vi "SupportedMeasurementType.vi"(8 "error in (no error)":errorcluster, 11 "ChromaAcLoad in":refnum<class "ChromaAcLoad.lvclass">) -> (0 "error out":errorcluster, 3 "ChromaAcLoad out":refnum<class "ChromaAcLoad.lvclass">)   [LabVIEW 2018, in "AcPwrPlugins.lvlib" / "ChromaAcLoad.lvclass"]
doc: "This VI checks if Measurment Types selected are capable by the instrument based on the instruments configuration."
uses:
  ChromaAcLoad.lvclass
  TypeDefs/MeasurementType.ctl
  <vilib>/Utility/error.llb/Error Cluster From Error Code.vi
  <vilib>/ErrorRing/Error Ring.xnode
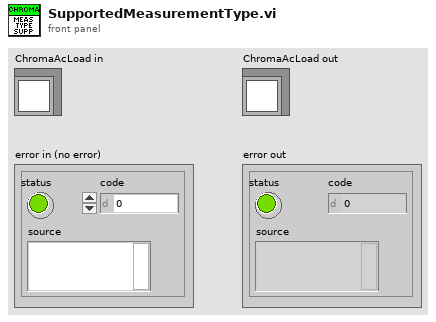
[diagram p1: front panel]
types:
  T1 = typedef "AcPwrPlugins.lvlib/ChromaAcLoad.lvclass/Device(s)Settings.ctl" = cluster{"Configuration Mode":enum16{"Constant Voltage (DC)", "Constant Power (DC)", "Constant Power (AC)", "Constant Current (DC)", "Constant Current (AC)", "Constant Resistance (DC)", "Constant Resistance (AC)", "Rectified Mode (DC)", "Inrush (AC)", "RLC CP (AC)", "RLC (AC)"}, "Phases":cluster{"Handle":string, "Name":string, "Phase Select":i32, "Instrument Options":string, "id query (T)":bool, "reset device (T)":bool, "Load Short Circuited":bool, "Line Synchronization":bool, "Load Current (A/Arms)":dbl, "Load Voltage (V/Vrms)":dbl, "Load Power (W)":dbl, "Load Resistance (Ohms)":dbl, "Load Current Peak Limit (A)":dbl, "Load Current Limit (A/Arms)":dbl, "Load Power Limit (W)":dbl, "Synch Frequency (Hz)":dbl, "Priority":enum16{"CF Only", "PF Only", "Both (CF)", "Both (PF)"}, "Crest Factor":dbl, "Power Factor":dbl, "Slew Rate":cluster{"Rise Slew Rate (A/ms)":i32, "Fall Slew Rate (A/ms)":i32}, "LC/RLC Mode":cluster{"Capacitance (uF)":i32, "Inductance (uH)":i32, "Series Resistance (Ohm)":dbl, "Parallel Resistance (Ohm)":dbl}, "Timing":cluster{"TimingOn":enum16{""}, "Hours":u32, "Minutes":u32, "Seconds":dbl, "CutoffVoltage":dbl}, "Connected":bool}[], "MeasName":string}
  T2 = typedef "AcPwrPlugins.lvlib/ChromaAcLoad.lvclass/Measurements.ctl" = cluster{"Handle":string, "Name":string, "Enabled":bool, "Measurement Value":dbl, "Hold Peak Current Measurement":bool, "btnMeasFetch":bool, "ProtectionStatusString":string, "Measurement Type":T3}[]
  T3 = typedef "AcPwrPlugins.lvlib/ChromaAcLoad.lvclass/MeasurementType.ctl" = enum16{"Voltage (Vrms or V)", "Current (Arms or A)", "Power (W)", "Peak Voltage (V)", "Peak Current (A)", "Peak Power (W)", "Frequency (Hz)", "Resistance (Ohms)", "Voltage Overshoot (V)", "Positive Peak Current (A)", "Voltage Undershoot (V)", "Negative Peak Current (A)", "Apparent Power (VA)", "Reacitive Power (VAR)", "Voltage THD", "Power Factor", "Current's Crest Factor"}
  T4 = cluster{"Handle":string, "Name":string, "Phase Select":i32, "Instrument Options":string, "id query (T)":bool, "reset device (T)":bool, "Load Short Circuited":bool, "Line Synchronization":bool, "Load Current (A/Arms)":dbl, "Load Voltage (V/Vrms)":dbl, "Load Power (W)":dbl, "Load Resistance (Ohms)":dbl, "Load Current Peak Limit (A)":dbl, "Load Current Limit (A/Arms)":dbl, "Load Power Limit (W)":dbl, "Synch Frequency (Hz)":dbl, "Priority":enum16{"CF Only", "PF Only", "Both (CF)", "Both (PF)"}, "Crest Factor":dbl, "Power Factor":dbl, "Slew Rate":cluster{"Rise Slew Rate (A/ms)":i32, "Fall Slew Rate (A/ms)":i32}, "LC/RLC Mode":cluster{"Capacitance (uF)":i32, "Inductance (uH)":i32, "Series Resistance (Ohm)":dbl, "Parallel Resistance (Ohm)":dbl}, "Timing":cluster{"TimingOn":enum16{""}, "Hours":u32, "Minutes":u32, "Seconds":dbl, "CutoffVoltage":dbl}, "Connected":bool}[]
  T5 = enum16{"Constant Voltage (DC)", "Constant Power (DC)", "Constant Power (AC)", "Constant Current (DC)", "Constant Current (AC)", "Constant Resistance (DC)", "Constant Resistance (AC)", "Rectified Mode (DC)", "Inrush (AC)", "RLC CP (AC)", "RLC (AC)"}
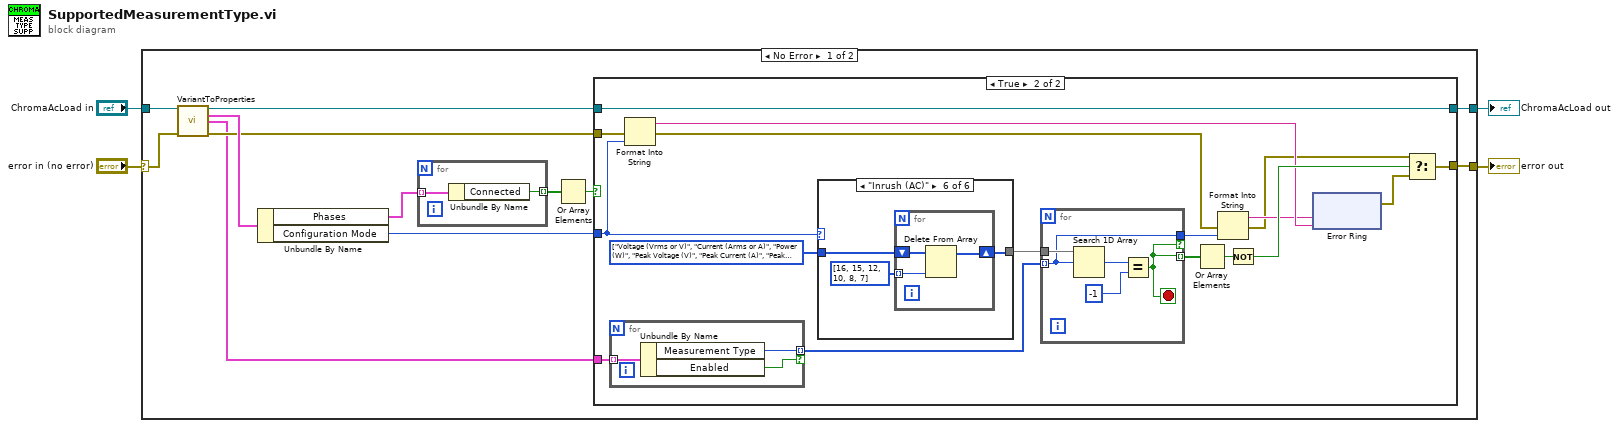
[diagram p0: block diagram]
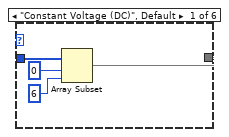
[diagram p3: hidden frame]
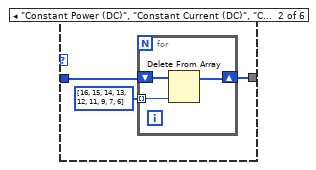
[diagram p4: hidden frame]
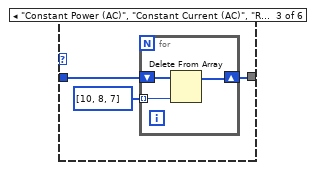
[diagram p5: hidden frame]
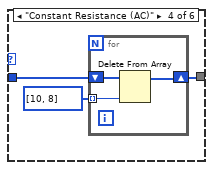
[diagram p6: hidden frame]
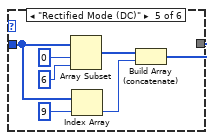
[diagram p7: hidden frame]
diagram:
  n1 = case shown="No Error" "error in (no error)" {
    selector: "error in (no error)" -> [w15 w90]
    tunnel: [w14 w90] -> w3
    tunnel: [w6 w89] -> w1
    tunnel: "ChromaAcLoad in" -> [w16 w89]
    frame No Error {
      n2 = call "VariantToProperties.vi"("ChromaAcLoad"=w16, "error in (no error)"=w15) -> ("ChromaAcLoad"=w7:refnum<class "ChromaAcLoad.lvclass">, "Device Properties"=w9:T1, "Meas"=w5:T2, "error out"=w8:errorcluster)  [unwired: 7 in, 3 out]
      n3 = Unbundle By Name(w9) -> ("Phases"=w12:T4, "Configuration Mode"=w13:T5)
      n4 = for {
        tunnel: w12 -> [w18] mode=indexing
        tunnel: [w17] -> w11 mode=indexing
        n5 = Unbundle By Name(w18) -> ("Connected"=w17:bool)
      }
      n6 = Or Array Elements(Boolean array=w11) -> (logical OR=w10:bool)
      n7 = case shown="True" w10 {
        tunnel: w5 -> [_ w36]
        tunnel: [w20 w29] -> w14
        tunnel: w13 -> [_ w28]
        tunnel: w8 -> [w20 w22]
        tunnel: w7 -> [w19 w21]
        tunnel: [w19 w21] -> w6
        frame False {
        }
        frame True {
          w37 = T3[] [enum."Voltage (Vrms or V)", enum."Current (Arms or A)", enum."Power (W)", enum."Peak Voltage (V)", enum."Peak Current (A)", enum."Peak Power (W)", enum."Frequency (Hz)", enum."Resistance (Ohms)", enum."Voltage Overshoot (V)", enum."Positive Peak Current (A)", enum."Voltage Undershoot (V)", enum."Negative Peak Current (A)", enum."Apparent Power (VA)", enum."Reacitive Power (VAR)", enum."Voltage THD", enum."Power Factor", enum."Current's Crest Factor"] items=["Voltage (Vrms or V)", "Current (Arms or A)", "Power (W)", "Peak Voltage (V)", "Peak Current (A)", "Peak Power (W)", "Frequency (Hz)", "Resistance (Ohms)", "Voltage Overshoot (V)", "Positive Peak Current (A)", "Voltage Undershoot (V)", "Negative Peak Current (A)", "Apparent Power (VA)", "Reacitive Power (VAR)", "Voltage THD", "Power Factor", "Current's Crest Factor"] ("MeasurementTypeArray")
          n8 = for {
            tunnel: w36 -> [w88] mode=indexing
            tunnel: [w87] -> w35 mode=indexing if=w86
            n9 = Unbundle By Name(w88) -> ("Measurement Type"=w87:T3, "Enabled"=w86:bool)
          }
          n10 = Format Into String(error in=w22, w28) -> (resulting string=w27:string, error out=w24:errorcluster)  [unwired: 2 in]
          n11 = case shown="\"Inrush (AC)\"" w28 {
            tunnel: w37 -> [w41 w43 w50 w55 w64 w68]
            tunnel: [w38 w42 w49 w54 w61 w67] -> w34
            frame "Constant Voltage (DC)", Default {
              n12 = Array Subset(array=w41, index=0, length=6) -> (w38:T3[])
            }
            frame "Constant Power (DC)", "Constant Current (DC)", "Constant Resistance (DC)" {
              n13 = for {
                shift-right: [w46] -> w42
                shift-left: w43 -> [w47]
                tunnel: i32[] [16, 15, 14, 13, 12, 11, 9, 7, 6] -> [w45] mode=indexing
                n14 = Delete From Array(array=w47, index=w45) -> (array with subset deleted=w46:T3[])  [unwired: 1 in, 1 out]
              }
            }
            frame "Constant Power (AC)", "Constant Current (AC)", "RLC CP (AC)", "RLC (AC)" {
              n15 = for {
                shift-right: [w52] -> w49
                shift-left: w50 -> [w53]
                tunnel: i32[] [10, 8, 7] -> [w51] mode=indexing
                n16 = Delete From Array(array=w53, index=w51) -> (array with subset deleted=w52:T3[])  [unwired: 1 in, 1 out]
              }
            }
            frame "Constant Resistance (AC)" {
              n17 = for {
                shift-right: [w58] -> w54
                shift-left: w55 -> [w59]
                tunnel: i32[] [10, 8] -> [w57] mode=indexing
                n18 = Delete From Array(array=w59, index=w57) -> (array with subset deleted=w58:T3[])  [unwired: 1 in, 1 out]
              }
            }
            frame "Rectified Mode (DC)" {
              n19 = Array Subset(array=w64, index=0, length=6) -> (w63:T3[])
              n20 = Index Array(array=w64, index=9) -> (element=w62:T3)
              n21 = Build Array (concatenate)(w63, w62) -> (w61:T3[])
            }
            frame "Inrush (AC)" {
              n22 = for {
                shift-right: [w71] -> w67
                shift-left: w68 -> [w72]
                tunnel: i32[] [16, 15, 12, 10, 8, 7] -> [w70] mode=indexing
                n23 = Delete From Array(array=w72, index=w70) -> (array with subset deleted=w71:T3[])  [unwired: 1 in, 1 out]
              }
            }
          }
          n24 = for {
            tunnel: w35 -> [w82] mode=indexing
            tunnel: w34 -> [w85]
            tunnel: [w82] -> w26 if=w81
            tunnel: [w81] -> w33 mode=indexing
            stop <- w81 stop-if-true
            n25 = Search 1D Array(1D array=w85, element=w82) -> (index of element=w84:i32)  [unwired: 1 in]
            n26 = Equal?(x=w84, y=-1) -> (x = y?=w81:bool)
          }
          n27 = Or Array Elements(Boolean array=w33) -> (logical OR=w32:bool)
          n28 = Format Into String(error in=w24, w26) -> (resulting string=w25:string, error out=w23:errorcluster)  [unwired: 2 in]
          n29 = Not(x=w32) -> (.not. x?=w31:bool)
          n30 = xnode "Error Ring"("parameter 0"=w25, "parameter 1"=w27) -> ("error out"=w30:errorcluster)
          n31 = Select(t=w23, s=w31, f=w30) -> (s? t:f=w29:errorcluster)
        }
      }
    }
    frame Error {
    }
  }
  "error out" <- w3
  "ChromaAcLoad out" <- w1
